vi "Window Direct Message.vi"(8 "error in (no error)":errorcluster, 10 "Message Cluster":T1, 11 "Chat Room Window in":refnum<class "Chat Room Window.lvclass">) -> (0 "error out":errorcluster, 3 "Chat Room Window out":refnum<class "Chat Room Window.lvclass">)   [LabVIEW 2020, in "Interface.lvlib" / "Chat Room Window.lvclass"]
uses:
  Chat Room Window.lvclass
  Application Control/Message.ctl
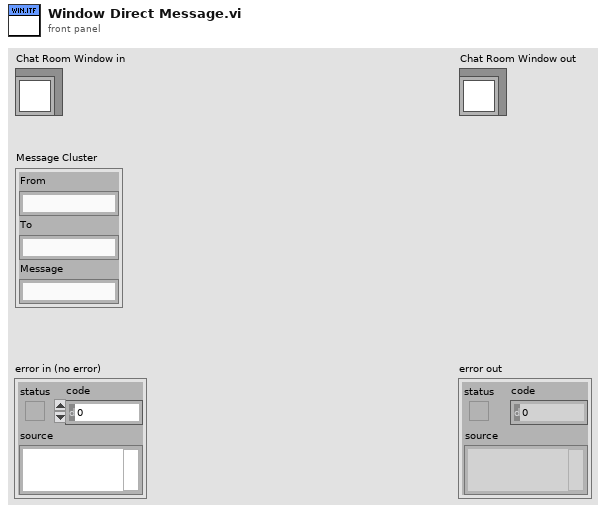
[diagram p1: front panel]
types:
  T1 = typedef "Message.ctl" = cluster{"From":string, "To":string, "Message":string}
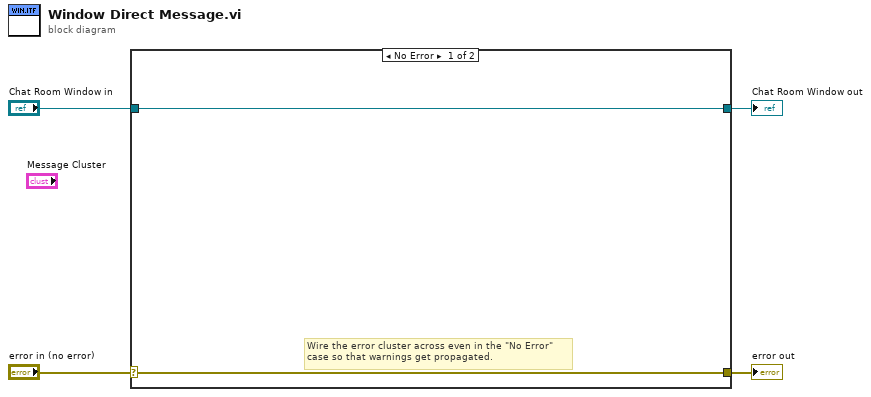
[diagram p0: block diagram]
diagram:
  n1 = case shown="No Error" "error in (no error)" {
    selector: "error in (no error)" -> [w5 w8]
    tunnel: [w5 w8] -> w3
    tunnel: [w6 w7] -> w1
    tunnel: "Chat Room Window in" -> [w6 w7]
    frame No Error {
      # "Wire the error cluster across even in the \"No Error\"\ncase so that warnings get propagated."
    }
    frame Error {
    }
  }
  "error out" <- w3
  "Chat Room Window out" <- w1
